vi "AutoMoveSubVI2.vi"() -> ()   [LabVIEW 2010]
uses:
  <vilib>/NXT/Subs/LVHSConnector.ctl
  <vilib>/NXT/Subs/MotorXNode.DC Motor Type.ctl
  <vilib>/NXT/HiTechnic/HiTechnic Controls/HiTechnic Port.ctl
  <vilib>/NXT/Block Support/NXT_InputPort.ctl
  <vilib>/NXT/NXTIO Xnodes/NXTIOXNode/NXTIO.xnode
  <vilib>/NXT/Subs/MotorXNode.2DCMotor.ctl
  <vilib>/NXT/NXTIO Xnodes/NXTIONodeSubVIs/TETRIX IO Move DC Motors.vi
panel:
  in  "Time":u32
  in  "index":i32
  in  "NXT 2":T1
  in  "DC Motor":T3
  in  "Power/Speed 2":i8
  in  "Power/Speed 1":i8
  out "NXT":T1
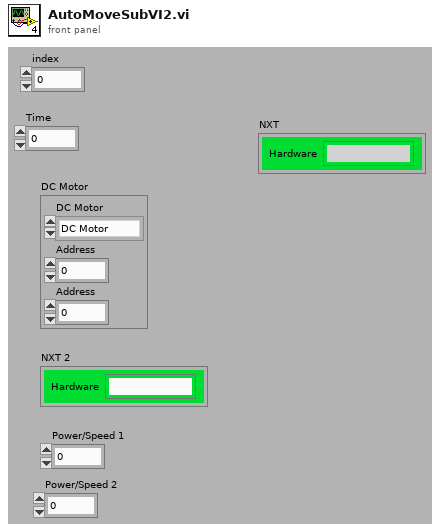
[diagram p1: front panel]
types:
  T1 = typedef "LVHSConnector.ctl" = cluster{"Hardware":string, "Flattened String":string}
  T2 = typedef "MotorXNode.DC Motor Type.ctl" = enum16{"DC Motor"}
  T3 = cluster{"DC Motor":T2, "Address":i16, "Address":i16}
  T4 = typedef "HiTechnic Port.ctl" = cluster{"Port":T5, "MUX Port":u8}
  T5 = typedef "NXT_InputPort.ctl" = u8
  T6 = cluster{"Direction (0-9)":i16, "Signal Strength (Array)":u8[]}
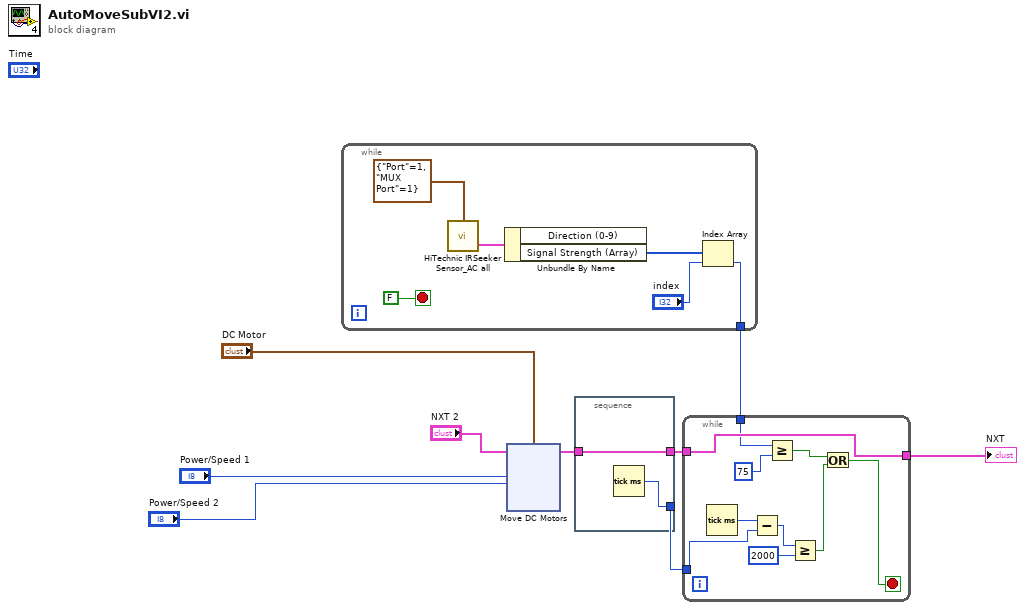
[diagram p0: block diagram]
diagram:
  n1 = while {
    tunnel: [w11] -> w1
    stop <- FALSE stop-if-true
    n2 = call <vilib>:"HiTechnic IRSeeker Sensor_AC all.vi"("Port/MUX"=T4 {"Port"=1, "MUX Port"=1}) -> ("All Info"=w14:T6)  [unwired: 2 in, 1 out]
    n3 = Unbundle By Name(w14) -> ("Signal Strength (Array)"=w13:u8[])  [unwired: 1 out]
    n4 = Index Array(array=w13, index="index") -> (element=w11:u8)
  }
  n5 = xnode "Move DC Motors"("Power/Speed 2"="Power/Speed 2", "Power/Speed 1"="Power/Speed 1", "Motors"="DC Motor", "NXT"="NXT 2") -> ("NXT"=w5:T1)
  n6 = stacked-sequence {
    tunnel: [w17] -> w4
    tunnel: w5 -> [w16]
    tunnel: [w16] -> w2
    frame #0 {
      n7 = Tick Count (ms)() -> (millisecond timer value=w17:u32)
    }
  }
  n8 = while {
    tunnel: w4 -> [w27]
    tunnel: w2 -> [w20]
    tunnel: [w20] -> w8
    tunnel: w1 -> [w19]
    stop <- w18 stop-if-true
    n9 = Tick Count (ms)() -> (millisecond timer value=w25:u32)
    n10 = Subtract(x=w25, y=w27) -> (x-y=w24:u32)
    n11 = Greater Or Equal?(x=w19, y=u8 75) -> (x >= y?=w22:bool)
    n12 = Greater Or Equal?(x=w24, y=u32 2000) -> (x >= y?=w21:bool)
    n13 = Or(x=w22, y=w21) -> (x .or. y?=w18:bool)
  }
  "NXT" <- w8
